vi "ReadEXCEL.vi"(8 "错误输入（无错误）":errorcluster, 9 "EXCEL 标签":string="Sheet1", 10 "路径":path) -> (0 "错误输出":errorcluster, 1 "数据":string[][](array[string]))   [LabVIEW 2014]
panel:
  in  "数组":string[][](array[string])
  in  "Excel._Worksheet":refnum<k7>
  in  "Excel._Application":refnum<k7>
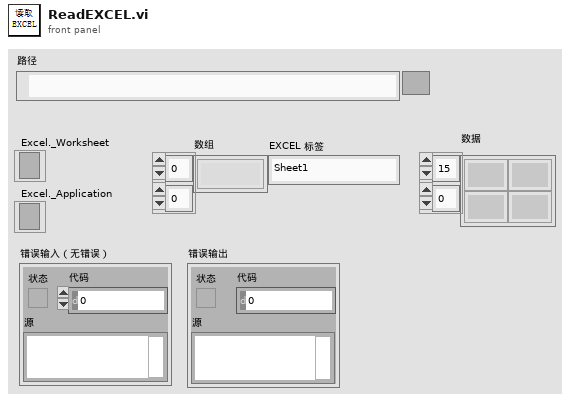
[diagram p1: front panel]
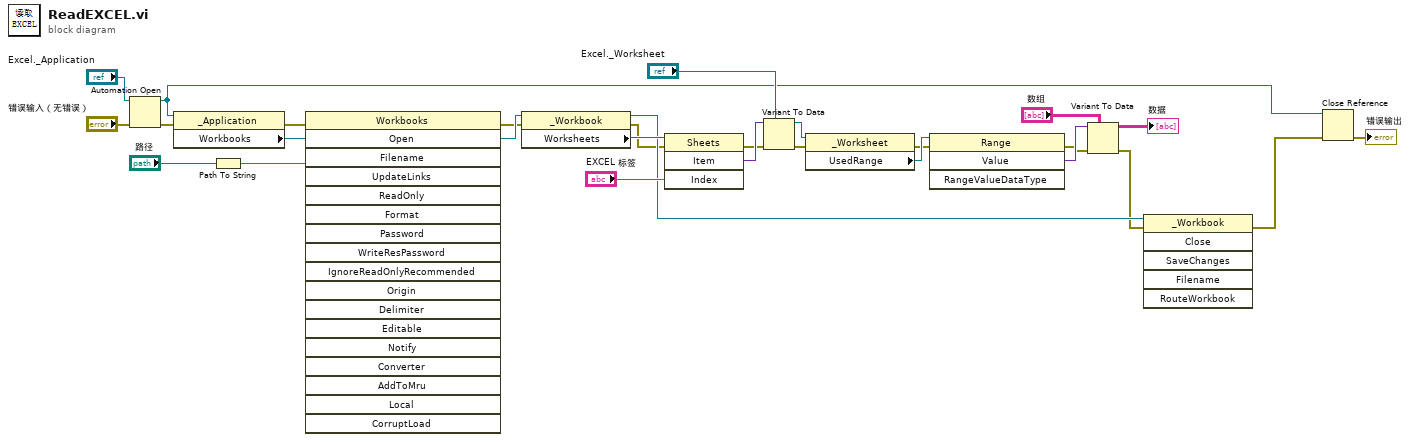
[diagram p0: block diagram]
diagram:
  n1 = Automation Open(error in (no error)="错误输入（无错误）", Automation Refnum="Excel._Application") -> (Automation Refnum=w7:refnum<k7>, error out=w28:errorcluster)  [unwired: 2 out]
  n2 = property class="_Application"(reference=w7, error in=w28) -> (error out=w27:errorcluster, "Workbooks"=w10:refnum<k7>)  [unwired: 1 out]
  n3 = Path To String(path="路径") -> (string=w9:string)
  n4 = invoke class="Workbooks" method="Open"(reference=w10, error in=w27, "Filename"=w9) -> (error out=w25:errorcluster, "Open"=w26:refnum<k7>)  [unwired: 15 in, 16 out]
  n5 = property class="_Workbook"(reference=w26, error in=w25) -> (reference out=w8:refnum<k7>, error out=w1:errorcluster, "Worksheets"=w24:refnum<k7>)
  n6 = invoke class="Sheets" method="Item"(reference=w24, error in=w1, "Index"="EXCEL 标签") -> (error out=w21:errorcluster, "Item"=w23:variant)  [unwired: 1 in, 2 out]
  n7 = Variant To Data(error in=w21, type="Excel._Worksheet", Variant=w23) -> (data=w20:refnum<k7>, error out=w17:errorcluster)
  n8 = property class="_Worksheet"(reference=w20, error in=w17) -> (error out=w16:errorcluster, "UsedRange"=w19:refnum<k7>)  [unwired: 1 out]
  n9 = invoke class="Range" method="Value"(reference=w19, error in=w16) -> (error out=w15:errorcluster, "Value"=w18:variant)  [unwired: 2 in, 2 out]
  n10 = Variant To Data(error in=w15, type="数组", Variant=w18) -> (data=→"数据":string[][], error out=w5:errorcluster)
  n11 = invoke class="_Workbook" method="Close"(reference=w8, error in=w5) -> (error out=w6:errorcluster)  [unwired: 4 in, 5 out]
  n12 = Close Reference(reference=w7, error in (no error)=w6) -> (error out=→"错误输出":errorcluster)
